vi "Read Summary.vi"(8 "error in (no error)":errorcluster, 11 "Request in":refnum<class "Request.lvclass">) -> (0 "error out":errorcluster, 2 "Description":string, 3 "Request out":refnum<class "Request.lvclass">)   [LabVIEW 2015, in "Request.lvclass"]
uses:
  Request.lvclass
  Request.lvclass/Request.ctl
  SummaryJsonCluster.ctl
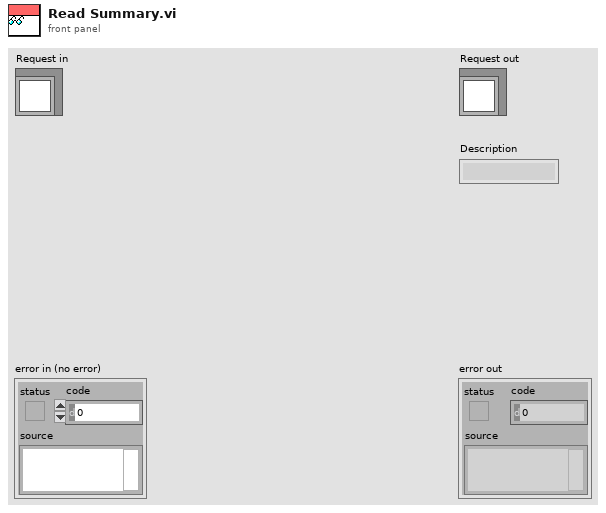
[diagram p1: front panel]
types:
  T1 = typedef "Request.lvclass/SummaryJsonCluster.ctl" = cluster{"RequestID":string, "EnlapsedTime":i32, "Description":string, "Alarm":bool}
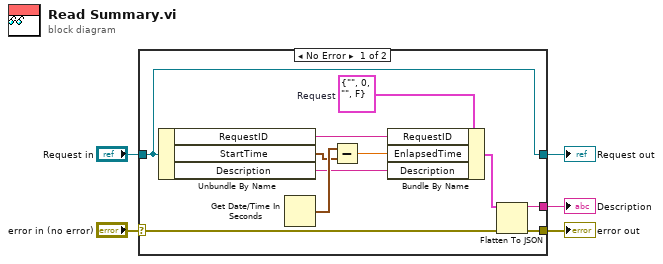
[diagram p0: block diagram]
diagram:
  n1 = case shown="No Error" "error in (no error)" {
    selector: "error in (no error)" -> [w15 w17]
    tunnel: [w14 w17] -> w4
    tunnel: [w11 w18] -> w2
    tunnel: "Request in" -> [w11 w18]
    tunnel: [w16 _] -> w1
    frame No Error {
      w12 = T1 {"RequestID"="", "EnlapsedTime"=0, "Description"="", "Alarm"=FALSE}  # Request
      n2 = Unbundle By Name(w11) -> ("RequestID"=w10:string, "StartTime"=w8:timestamp, "Description"=w6:string)
      n3 = Get Date/Time In Seconds() -> (seconds since 1Jan1904=w9:timestamp)
      n4 = Subtract(x=w9, y=w8) -> (x-y=w7:dbl)
      n5 = Bundle By Name(cluster=w12, "RequestID"=w10, "EnlapsedTime"=w7, "Description"=w6) -> (w13:T1)
      n6 = Flatten To JSON(anything=w13, error in (no error)=w15) -> (JSON string=w16:string, 11:w14:errorcluster)  [unwired: 1 in]
    }
    frame Error {
    }
  }
  "error out" <- w4
  "Request out" <- w2
  "Description" <- w1
